vi "Set DG535 for LED.vi"(7 "amplitude":dbl=1.0 min=-3.0 max=4.0 format="%.2f", 8 "error in":errorcluster, 9 "Delay (ms)":dbl, 10 "Pulse length (ms)":dbl, 11 "GPIB address":string="15") -> (0 "error out":errorcluster)   [LabVIEW 2013]
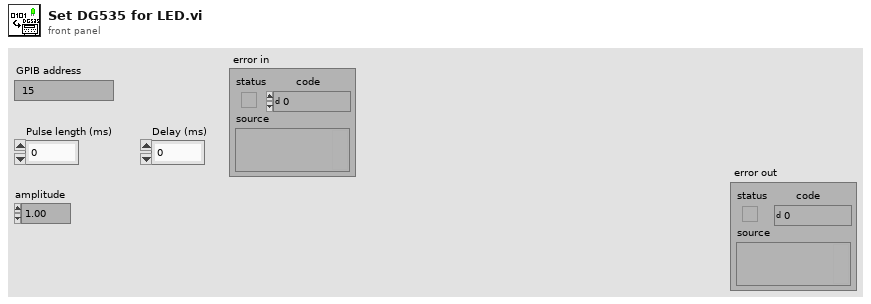
[diagram p1: front panel]
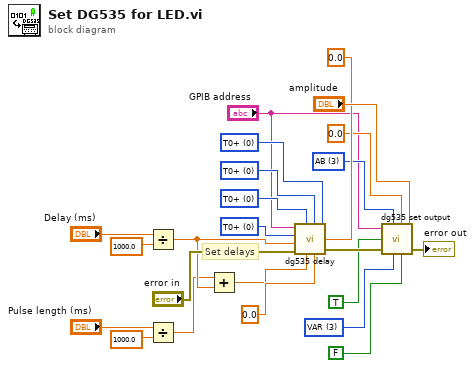
[diagram p0: block diagram]
diagram:
  w9 = 3 items=["TTL", "NIM", "ECL", "VAR"] ("mode")
  w11 = u16 3 items=["T0", "A", "B", "AB", "C", "D", "CD"] ("output")
  w18 = u32 0 items=["T0+", "A+", "B+", "C+"] ("D=")
  w19 = u32 0 items=["T0+", "A+", "B+", "D+"] ("C=")
  w20 = u32 0 items=["T0+", "A+", "C+", "D+"] ("B=")
  w21 = u32 0 items=["T0+", "B+", "C+", "D+"] ("A=")
  # "Set delays"
  n1 = Divide(x="Delay (ms)", y=1000.0) -> (x/y=w4:dbl)
  n2 = Divide(x="Pulse length (ms)", y=1000.0) -> (x/y=w3:dbl)
  n3 = Add(x=w3, y=w4) -> (x+y=w2:dbl)
  n4 = call "dg535 delay.vi"("C"=0.0, "D"=0.0, "D="=w18, "C="=w19, "B"=w2, "error in"="error in", "A"=w4, "B="=w20, "A="=w21, "GPIB address"="GPIB address") -> ("error out"=w13:errorcluster)
  n5 = call "dg535 set output.vi"("GPIB address"="GPIB address", "output"=w11, "set"=TRUE, "error in"=w13, "mode"=w9, "offset"=0.0, "amplitude"="amplitude", "load"=FALSE) -> ("error out"=→"error out":errorcluster)  [unwired: 1 in]
